vi "Station_Wise_Enable_Disable_Alalrm_Indi.vi"(6 "Autonomous Check Points Press":refnum<vi>, 8 "error in (no error)":errorcluster, 10 "?":T1={"Product List"=[], "SQL reference"=refnum, "Indicator refrence"=[], "Station Number"=[], "Shift Time stamp"=[timestamp(3597615000 s since 1904-01-01), timestamp(3597658199 s since 1904-01-01), timestamp(3597658200 s since 1904-01-01), timestamp(3597614999 s since 1904-01-01), timestamp(3597589800 s since 1904-01-01), timestamp(3597589800 s since 1904-01-01)], "Com Status Station"=[], "ALARAM INDICATOR REF"=[], "Reading"=[], "Read Parameteres"=[], "Station Name"=[], "Oven Read Parameteres"=[]} {"Shift Time stamp" format="%<%X>T"}, 11 "Alarm array":refnum<vi>[](array[refnum])) -> (0 "error out":errorcluster, 3 "Valid Indicators":refnum<vi>[](array[refnum]))   [LabVIEW 2017]
doc: "This vi is used to diable the alarm indicators in Station_Wise_VI AND this vi is used to name the indicator with station names"
uses:
  Controls/station_wise_loop_data.ctl
  <vilib>/addons/database/Connection.llb/Conn ObjectReference.ctl
  <vilib>/addons/database/NI_Database_API.lvlib
panel:
  out "MACHINE 1":T3
  out "Display 1":T4
  # "Communication:-"
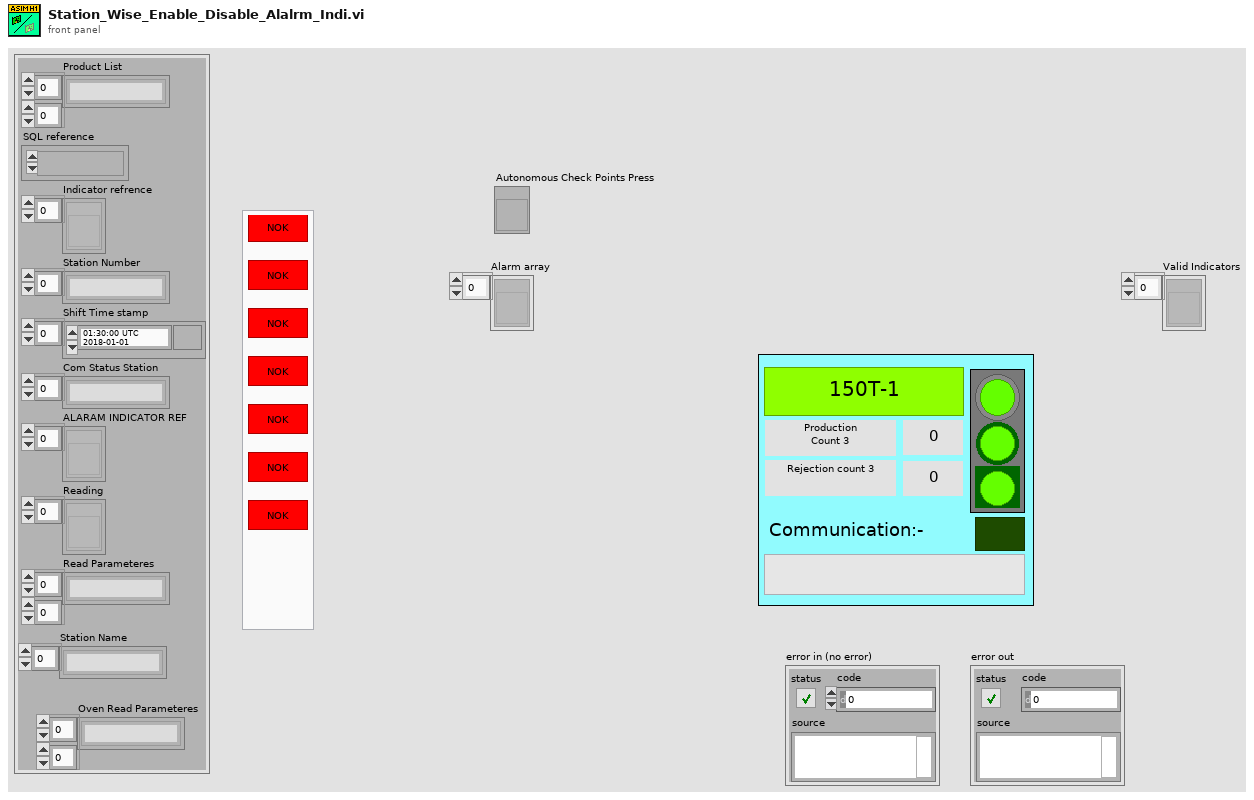
[diagram p1: front panel]
types:
  T1 = typedef "station_wise_loop_data.ctl" = cluster{"Product List":string[][], "SQL reference":T2, "Indicator refrence":refnum<vi>[], "Station Number":string[], "Shift Time stamp":timestamp[], "Com Status Station":string[], "ALARAM INDICATOR REF":refnum<vi>[], "Reading":refnum<vi>[], "Read Parameteres":string[][], "Station Name":string[], "Oven Read Parameteres":string[][]}
  T2 = typedef "NI_Database_API.lvlib/Conn ObjectReference.ctl" = refnum<k1>
  T3 = cluster{"M1.1":bool, "M1.1 2":bool, "M1.1 3":bool, "M1.1 4":bool, "M1.1 5":bool, "M1.1 6":bool, "M1.1 7":bool, "M1.1 8":bool, "M1.1 9":bool}
  T4 = cluster{"Status 10":cluster{"S":bool, "l":bool, "M":bool, "Q":bool, "P":bool}, "Station Name":bool, "Production\nCount 3":i32, "Rejection count 3":i32, "String Indicator 3":bool, "Product code 10":string}
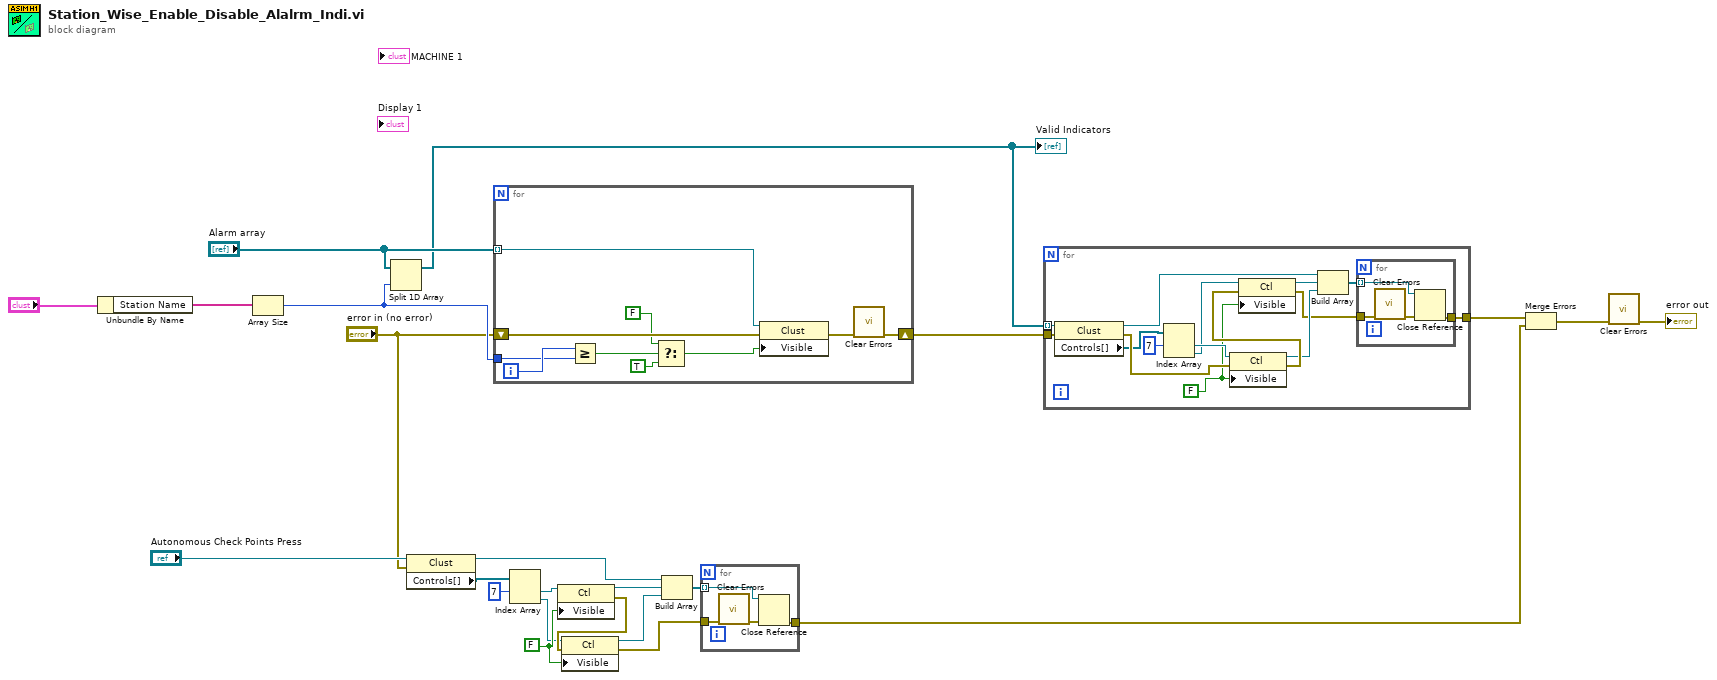
[diagram p0: block diagram]
diagram:
  w13 = FALSE
  n1 = Unbundle By Name("?") -> ("Station Name"=w19:string[])
  n2 = Array Size(array=w19) -> (size(s)=w22:i32)
  n3 = Split 1D Array(array="Alarm array", index=w22) -> (first subarray=w18:refnum<vi>[])  [unwired: 1 out]
  "Valid Indicators" <- w18
  n4 = property on="Property Node" class="Clust"(reference="Autonomous Check Points Press", error in="error in (no error)") -> (reference out=w7:refnum<vi>, "Controls[]"=w14:refnum<vi>[])  [unwired: 1 out]
  n5 = for {
    shift-right: [w31] -> w16
    shift-left: "error in (no error)" -> [w33]
    tunnel: "Alarm array" -> [w24] mode=indexing
    tunnel: w22 -> [w29]
    i -> [w30]
    n6 = Greater Or Equal?(x=w30, y=w29) -> (x >= y?=w28:bool)
    n7 = Select(t=FALSE, s=w28, f=TRUE) -> (s? t:f=w25:bool)
    n8 = property on="Property Node" class="Clust"(reference=w24, error in=w33, "Visible"=w25) -> (error out=w32:errorcluster)  [unwired: 1 out]
    n9 = call <vilib>:"Clear Errors.vi"("error in (no error)"=w32) -> ("error out"=w31:errorcluster)  [unwired: 5 in, 1 out]
  }
  n10 = Index Array(array=w14, index #1=7 ("index")) -> (element #1=w11:refnum<vi>, element #2=w10:refnum<vi>)  [unwired: 1 in]
  n11 = property class="Ctl"(reference=w11, "Visible"=w13) -> (reference out=w8:refnum<vi>, error out=w12:errorcluster)  [unwired: 1 in]
  n12 = property class="Ctl"(reference=w10, error in=w12, "Visible"=w13) -> (reference out=w5:refnum<vi>, error out=w6:errorcluster)
  n13 = Build Array(w7, w8, w5) -> (w9:refnum<vi>[])
  n14 = for {
    tunnel: w9 -> [w36] mode=indexing
    tunnel: [w35] -> w1
    tunnel: w6 -> [w34]
    n15 = call <vilib>:"Clear Errors.vi"("error in (no error)"=w34) -> ("error out"=w37:errorcluster)  [unwired: 5 in, 1 out]
    n16 = Close Reference(reference=w36, error in (no error)=w37) -> (error out=w35:errorcluster)
  }
  n17 = for {
    tunnel: w18 -> [w50] mode=indexing
    tunnel: [w40] -> w17
    tunnel: w16 -> [w38]
    w47 = FALSE ("Tabs Visible?")
    n18 = property on="Property Node" class="Clust"(reference=w50, error in=w38) -> (reference out=w39:refnum<vi>, error out=w52:errorcluster, "Controls[]"=w51:refnum<vi>[])
    n19 = Index Array(array=w51, index #1=7 ("index")) -> (element #1=w49:refnum<vi>, element #2=w46:refnum<vi>)  [unwired: 1 in]
    n20 = property class="Ctl"(reference=w49, error in=w52, "Visible"=w47) -> (reference out=w43:refnum<vi>, error out=w48:errorcluster)
    n21 = property class="Ctl"(reference=w46, error in=w48, "Visible"=w47) -> (reference out=w42:refnum<vi>, error out=w41:errorcluster)
    n22 = Build Array(w39, w42, w43) -> (w44:refnum<vi>[])
    n23 = for {
      tunnel: w44 -> [w55] mode=indexing
      tunnel: w41 -> [w54]
      tunnel: [w53] -> w40
      n24 = call <vilib>:"Clear Errors.vi"("error in (no error)"=w54) -> ("error out"=w56:errorcluster)  [unwired: 5 in, 1 out]
      n25 = Close Reference(reference=w55, error in (no error)=w56) -> (error out=w53:errorcluster)
    }
  }
  n26 = Merge Errors(w17, w1) -> (w2:errorcluster)
  n27 = call <vilib>:"Clear Errors.vi"("error in (no error)"=w2) -> ("error out"=→"error out":errorcluster)  [unwired: 5 in, 1 out]
